vi "AbortGeneration.vi"(8 "error in (no error)":errorcluster, 11 "NiPxi6733 in":refnum<class "NiPxi6733.lvclass">) -> (0 "error out":errorcluster, 3 "NiPxi6733 out":refnum<class "NiPxi6733.lvclass">)   [LabVIEW 2018, in "FgenPlugins.lvlib" / "NiPxi6733.lvclass"]
uses:
  NiPxi6733.lvclass
  X:/Projects/PMUCal/Modules/FGen/FgenPlugins/FgenPluginBaseClass/FgenPluginsBase.lvclass
  FgenPluginBaseClass/FgenPluginsBase.lvclass/FgenPluginsBase.ctl
  MemberClasses/FunctionBaseClass/FunctionBase.lvclass/FunctionBase.ctl
  <vilib>/DAQmx/write.llb/DAQmx Write (Analog 1D Wfm NChan NSamp).vi
  FgenPluginBaseClass/Accessors/Read Channels.vi
  FgenPluginBaseClass/Accessors/Read FunctionClass.vi
  MemberClasses/FunctionBaseClass/Accessors/Read Waveforms.vi
  <vilib>/DAQmx/miscellaneous.llb/DAQmx Fill In Error Info.vi
  MemberClasses/FunctionBaseClass/FunctionBase.lvclass
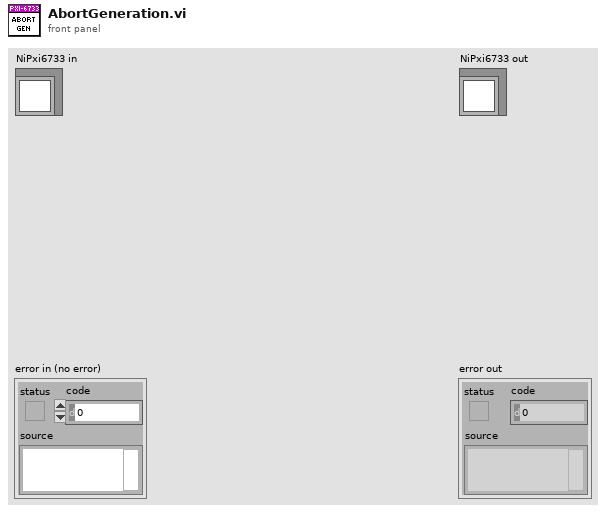
[diagram p1: front panel]
types:
  T1 = typedef "FgenPlugins.lvlib/Channel.ctl" = cluster{"Name":string, "Enabled":bool, "Operation":enum16{"Continuous", "Burst"}, "Impedance (50)":dbl, "Handle":string, "Connected":bool, "Mode (Function)":enum16{"Function", "Arbitrary", "Sequence"}}
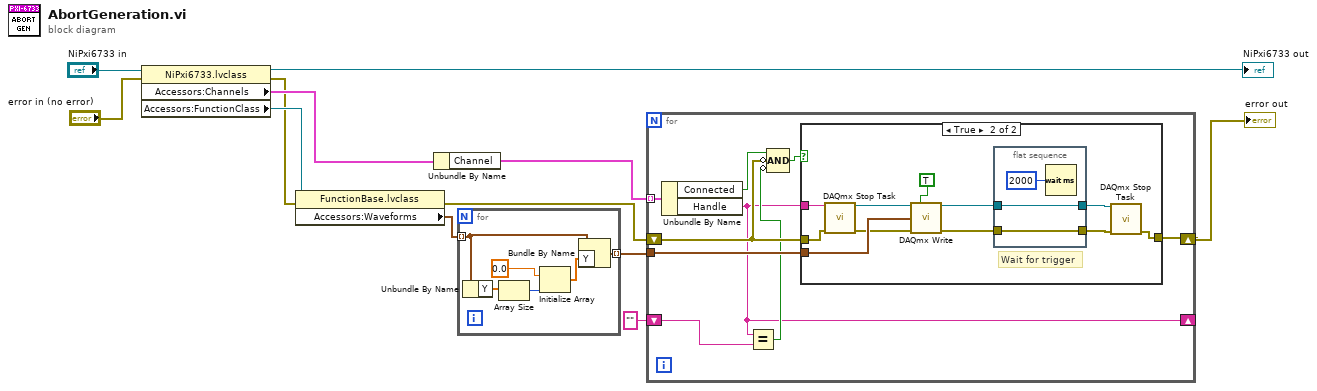
[diagram p0: block diagram]
diagram:
  n1 = property class="NiPxi6733.lvclass"(reference="NiPxi6733 in", error in="error in (no error)") -> (reference out=→"NiPxi6733 out":refnum<class "NiPxi6733.lvclass">, error out=w5:errorcluster, "Accessors:Channels"=w10:cluster{"Count":u16, "Channel":T1[]}, "Accessors:FunctionClass"=w9:refnum<class "FunctionBase.lvclass">)
  n2 = property class="FunctionBase.lvclass"(reference=w9, error in=w5) -> (error out=w4:errorcluster, "Accessors:Waveforms"=w8:waveform(dbl)[])  [unwired: 1 out]
  n3 = Unbundle By Name(w10) -> ("Channel"=w6:T1[])
  n4 = for {
    tunnel: w8 -> [w17] mode=indexing
    tunnel: [w18] -> w7 mode=indexing
    n5 = Unbundle By Name(w17) -> ("Y"=w16:dbl[])
    n6 = Array Size(array=w16) -> (size(s)=w14:i32)
    n7 = Initialize Array(0.0, w14) -> (w15:dbl[])
    n8 = Bundle By Name(cluster=w17, "Y"=w15) -> (w18:waveform(dbl))
  }
  n9 = for {
    tunnel: w6 -> [w27] mode=indexing
    tunnel: w7 -> [w26]
    shift-right: [w22] -> w2
    shift-left: w4 -> [w24]
    shift-right: [w19] -> _
    shift-left: "" ("Handle") -> [w21]
    n10 = Unbundle By Name(w27) -> ("Connected"=w25:bool, "Handle"=w19:string)
    n11 = Equal?(x=w19, y=w21) -> (x = y?=w20:bool)
    n12 = Compound Arithmetic op=AND(w25, invert w24, invert w20) -> (w23:bool)
    n13 = case shown="True" w23 {
      tunnel: w26 -> [_ w38]
      tunnel: w24 -> [w28 w36]
      tunnel: [w28 w33] -> w22
      tunnel: w19 -> [_ w37]
      frame False {
      }
      frame True {
        # "Wait for trigger"
        n14 = call <vilib>:"DAQmx Stop Task.vi"("task/channels in"=w37, "error in"=w36) -> ("task out"=w34:refnum<k21>, "error out"=w35:errorcluster)  [unwired: 12 in]
        n15 = call-poly <vilib>:"DAQmx Write.vi"("task/channels in"=w34, "auto start"=TRUE, "data"=w38, "error in"=w35) -> ("task out"=w32:refnum<k21>, "error out"=w29:errorcluster)  [unwired: 9 in, 1 out]
        n16 = flat-sequence {
          tunnel: [w42] -> w31
          tunnel: w32 -> [w42]
          tunnel: [w41] -> w30
          tunnel: w29 -> [w41]
          frame #0 {
            n17 = Wait (ms)(milliseconds to wait=u32 2000) -> ()  [unwired: 1 out]
          }
        }
        n18 = call <vilib>:"DAQmx Stop Task.vi"("task/channels in"=w31, "error in"=w30) -> ("error out"=w33:errorcluster)  [unwired: 12 in, 1 out]
      }
    }
  }
  "error out" <- w2
